vi "ep_Zoom Settings Configurator.vi"(8 "error in (no error)":errorcluster, 9 "block size":i32, 10 "fs":dbl, 11 "spectra settings":T2={"number of lines"=12501, "% overlap"=0.0, "maximum frequency [Hz]"=250.0}) -> (0 "error out":errorcluster, 3 "zoom FFT settings":T1 {"FFT settings"."window" items=["Rectangle"=0, "Hanning"=1, "Hamming"=2, "Blackman-Harris"=3, "Exact Blackman"=4, "Blackman"=5, "Flat Top"=6, "4 Term B-Harris "=7, "7 Term B-Harris"=8, "Low Sidelobe"=9, "Blackman Nuttall"=11, "Triangle"=30, "Bartlett-Hanning"=31, "Bohman"=32, "Parzen"=33, "Welch"=34, "Kaiser"=60, "Dolph-Chebyshev"=61, "Gaussian"=62]})   [LabVIEW 2014, in "NI_EP_Motor Monitoring.lvlib"]
uses:
  <vilib>/addons/Electrical Power/Motor Monitoring/NI_EP_Motor Monitoring.lvlib
  <vilib>/addons/Electrical Power/Motor Monitoring/subVIs/ep_Spectra Settings.ctl
  <vilib>/addons/Electrical Power/Motor Monitoring/subVIs/ep_Zoom FFT Settings.ctl
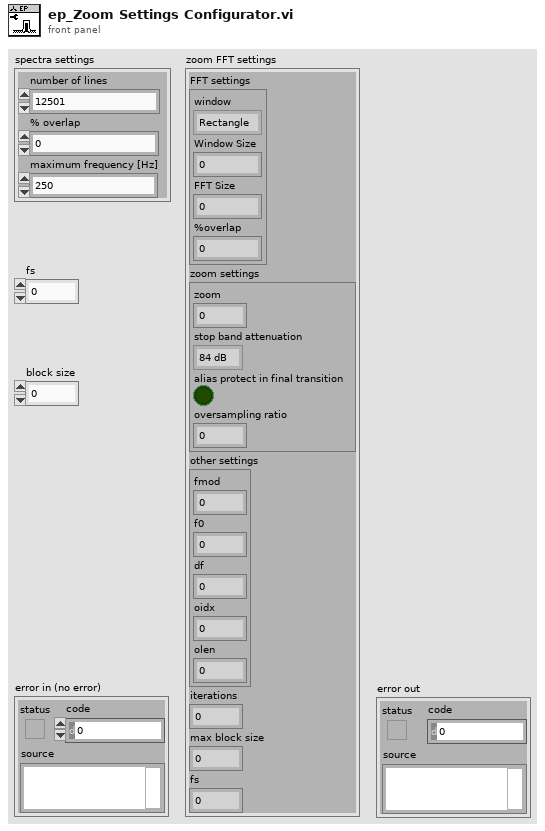
[diagram p1: front panel]
types:
  T1 = typedef "NI_EP_Motor Monitoring.lvlib/ep_Zoom FFT Settings.ctl" = cluster{"FFT settings":cluster{"window":u16, "Window Size":i32, "FFT Size":i32, "%overlap":dbl}, "zoom settings":cluster{"zoom":i32, "stop band attenuation":enum16{"84 dB", "96 dB", "120 dB"}, "alias protect in final transition":bool, "oversampling ratio":dbl}, "other settings":cluster{"fmod":dbl, "f0":dbl, "df":dbl, "oidx":i32, "olen":i32}, "iterations":i32, "max block size":i32, "fs":dbl}
  T2 = typedef "NI_EP_Motor Monitoring.lvlib/ep_Spectra Settings.ctl" = cluster{"number of lines":i32, "% overlap":dbl, "maximum frequency [Hz]":dbl}
  T3 = cluster{"fmod":dbl, "f0":dbl, "df":dbl, "oidx":i32, "olen":i32}
  T4 = cluster{"window":u16, "Window Size":i32, "FFT Size":i32, "%overlap":dbl}
  T5 = cluster{"zoom":i32, "stop band attenuation":enum16{"84 dB", "96 dB", "120 dB"}, "alias protect in final transition":bool, "oversampling ratio":dbl}
  T6 = enum16{"None ", "Hanning", "Hamming", "Blackman-Harris", "Exact Blackman", "Blackman", "Flat Top", "4 Term B-Harris ", "7 Term B-Harris", "Low Sidelobe"}
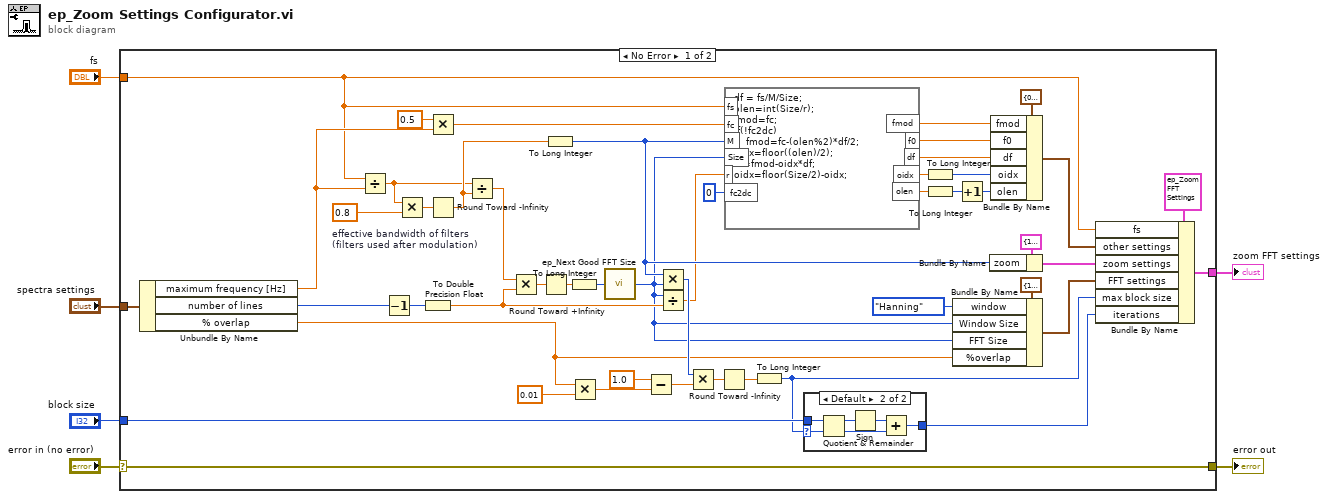
[diagram p0: block diagram]
diagram:
  n1 = case shown="No Error" "error in (no error)" {
    selector: "error in (no error)" -> [w54 w63]
    tunnel: "spectra settings" -> [w55 _]
    tunnel: [w54 w63] -> w3
    tunnel: "fs" -> [w8 _]
    tunnel: "block size" -> [w33 _]
    tunnel: [w11 _] -> w1
    frame No Error {
      w40 = 0.8  # effective bandwidth of filters (filters used after modulation)
      n2 = Unbundle By Name(w55) -> ("maximum frequency [Hz]"=w34:dbl, "number of lines"=w36:i32, "% overlap"=w29:dbl)
      n3 = Divide(x=w8, y=w34) -> (x/y=w41:dbl)
      n4 = Decrement(x=w36) -> (x-1=w38:i32)
      n5 = Multiply(x=w41, y=w40) -> (x*y=w46:dbl)
      n6 = To Double Precision Float(number=w38) -> (double precision float=w37:dbl)
      n7 = Multiply(x=0.5 ("y"), y=w34) -> (x*y=w28:dbl)
      n8 = Round Toward -Infinity ("Round To -Infinity")(1:w46) -> (0:w42:dbl)
      n9 = Divide(x=w41, y=w42) -> (x/y=w39:dbl)
      n10 = Multiply(x=w39, y=w37) -> (x*y=w45:dbl)
      n11 = Round Toward +Infinity ("Round To +Infinity")(x=w45) -> (ceil(x): smallest int >= x=w44:dbl)
      n12 = To Long Integer(number=w42) -> (32bit integer=w27:i32)
      n13 = To Long Integer(number=w44) -> (32bit integer=w43:i32)
      n14 = Multiply(x=w29, y=0.01) -> (x*y=w51:dbl)
      n15 = call <vilib>:"ep_Next Good FFT Size.vi"("FFT Size"=w43) -> ("least bigger good size"=w26:i32)
      n16 = Subtract(x=1.0, y=w51) -> (x-y=w50:dbl)
      n17 = Multiply(x=w27, y=w26) -> (x*y=w35:i32)
      n18 = Divide(x=w26, y=w37) -> (x/y=w25:dbl)
      n19 = Multiply(x=w35, y=w50) -> (x*y=w48:dbl)
      n20 = Round Toward -Infinity ("Round To -Infinity")(1:w48) -> (0:w49:dbl)
      n21 = formula code="df = fs/M/Size;\nolen=int(Size/r);\nfmod=fc;\nif(!fc2dc)\n    fmod=fc-(olen%2)*df/2;\noidx=floor((olen)/2);\nf0=fmod-oidx*df;\noidx=floor(Size/2)-oidx;"("fc"=w28, "M"=w27, "Size"=w26, "fs"=w8, "r"=w25, "fc2dc"=i16 0 ("input variable")) -> ("f0"=w22:dbl, "df"=w21:dbl, "oidx"=w20:dbl, "olen"=w19:dbl, "fmod"=w23:dbl)
      n22 = To Long Integer(number=w49) -> (32bit integer=w10:i32)
      n23 = case shown="Default" w10 {
        selector: w10 -> [w56 w61]
        tunnel: w33 -> [_ w62]
        tunnel: [w56 w58] -> w9
        frame 0 {
        }
        frame Default {
          n24 = Quotient & Remainder(x=w62, y=w61) -> (x-y*floor(x/y)=w60:i32, floor(x/y)=w57:i32)
          n25 = Sign(1:w60) -> (0:w59:i32)
          n26 = Add(x=w59, y=w57) -> (x+y=w58:i32)
        }
      }
      n27 = To Long Integer(number=w20) -> (32bit integer=w18:i32)
      n28 = To Long Integer(number=w19) -> (32bit integer=w17:i32)
      n29 = Bundle By Name(cluster=T4 {"window"=1, "Window Size"=1024, "FFT Size"=1024, "%overlap"=0.0} ("FFT settings"), "window"=T6."Hanning" ("FFT settings.window"), "Window Size"=w26, "FFT Size"=w26, "%overlap"=w29) -> (w12:T4)
      n30 = Increment(x=w17) -> (x+1=w16:i32)
      n31 = Bundle By Name(cluster=T5 {"zoom"=1, "stop band attenuation"=enum."120 dB", "alias protect in final transition"=FALSE, "oversampling ratio"=1.0} ("zoom settings"), "zoom"=w27) -> (w14:T5)
      n32 = Bundle By Name(cluster=T3 {"fmod"=0.0, "f0"=0.0, "df"=0.0, "oidx"=0, "olen"=0} ("zoom FFT settings"), "fmod"=w23, "f0"=w22, "df"=w21, "oidx"=w18, "olen"=w16) -> (w13:T3)
      n33 = Bundle By Name(cluster=T1 {"FFT settings"={"window"=0, "Window Size"=0, "FFT Size"=0, "%overlap"=0.0}, "zoom settings"={"zoom"=0, "stop band attenuation"=enum."84 dB", "alias protect in final transition"=FALSE, "oversampling ratio"=0.0}, "other settings"={"fmod"=0.0, "f0"=0.0, "df"=0.0, "oidx"=0, "olen"=0}, "iterations"=0, "max block size"=0, "fs"=0.0} ("zoom FFT settings"), "fs"=w8, "other settings"=w13, "zoom settings"=w14, "FFT settings"=w12, "max block size"=w10, "iterations"=w9) -> (w11:T1)
    }
    frame Error {
    }
  }
  "error out" <- w3
  "zoom FFT settings" <- w1
